vi "Read Status.vi"(8 "error in (no error)":errorcluster, 11 "Artifactory in":refnum<class "Artifactory.lvclass">) -> (0 "error out":errorcluster, 2 "Status":T1, 3 "Artifactory out":refnum<class "Artifactory.lvclass">)   [LabVIEW 2021, in "Artifactory.lvclass"]
uses:
  Artifactory.lvclass
  Artifactory.lvclass/Artifactory.ctl
  Status -- cluster.ctl
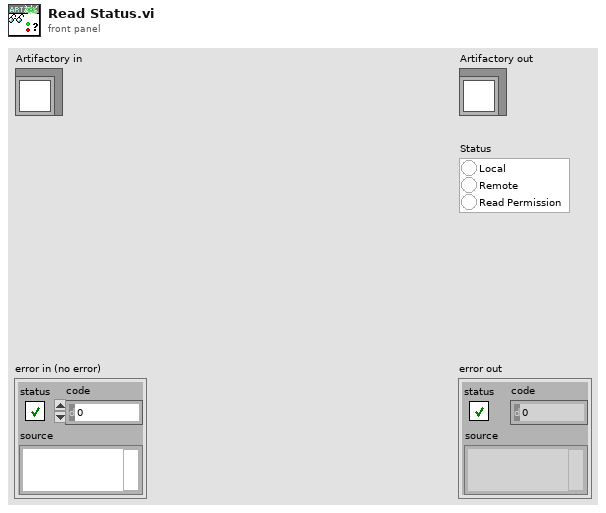
[diagram p1: front panel]
types:
  T1 = typedef "Artifactory.lvclass/Status -- cluster.ctl" = cluster{"Local":bool, "Remote":bool, "Read Permission":bool}
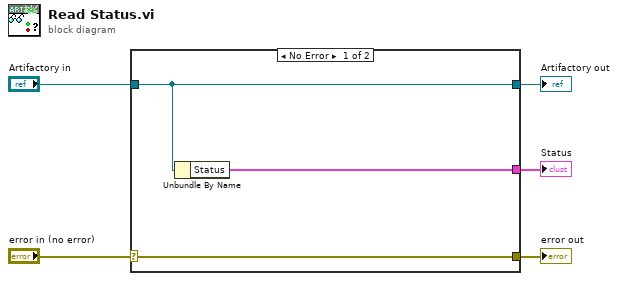
[diagram p0: block diagram]
diagram:
  n1 = case shown="No Error" "error in (no error)" {
    selector: "error in (no error)" -> [w8 w9]
    tunnel: [w8 w9] -> w4
    tunnel: [w7 w10] -> w2
    tunnel: "Artifactory in" -> [w7 w10]
    tunnel: [w6 _] -> w1
    frame No Error {
      n2 = Unbundle By Name(w7) -> ("Status"=w6:T1)
    }
    frame Error {
    }
  }
  "error out" <- w4
  "Artifactory out" <- w2
  "Status" <- w1
